vi "SupportedMetricsForHighLow.vi"() -> (3 "Supported Metrics":string[](array[string]))   [LabVIEW 2016, in "McsaAnalysisFunctions.lvlib"]
uses:
  <vilib>/addons/InsightCM/Utilities/Analysis/MCSA/McsaAnalysisFunctions.lvlib
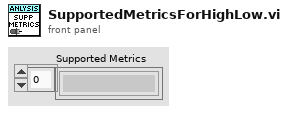
[diagram p1: front panel]
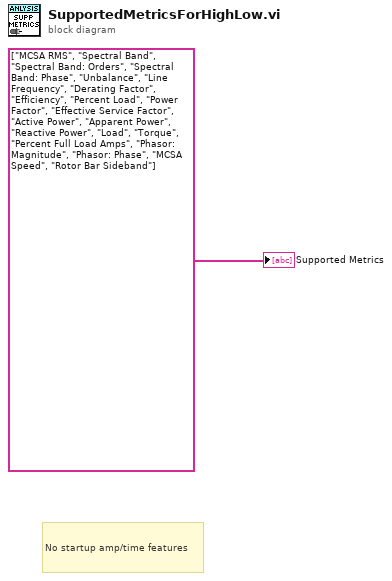
[diagram p0: block diagram]
diagram:
  # "No startup amp/time features"
  "Supported Metrics" <- string[] ["MCSA RMS", "Spectral Band", "Spectral Band: Orders", "Spectral Band: Phase", "Unbalance", "Line Frequency", "Derating Factor", "Efficiency", "Percent Load", "Power Factor", "Effective Service Factor", "Active Power", "Apparent Power", "Reactive Power", "Load", "Torque", "Percent Full Load Amps", "Phasor: Magnitude", "Phasor: Phase", "MCSA Speed", "Rotor Bar Sideband"] ("value")
